vi "Anzahl Span Eingänge Versa Hardware.vi"() -> (3 "Anzahl Span":i32)   [LabVIEW 2020, in "Linearisierung v2.lvlib" / "SpanEinstellungen.lvlib"]
uses:
  SpanEinstellungen.lvlib
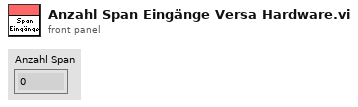
[diagram p1: front panel]
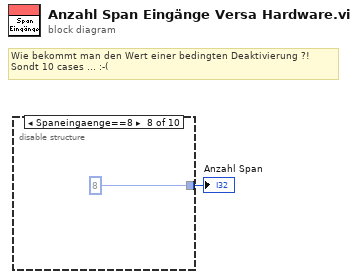
[diagram p0: block diagram]
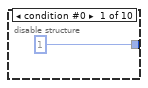
[diagram p2: hidden frame]
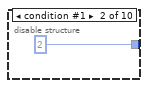
[diagram p3: hidden frame]
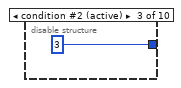
[diagram p4: hidden frame]
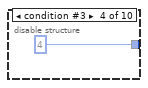
[diagram p5: hidden frame]
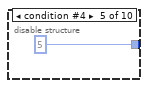
[diagram p6: hidden frame]
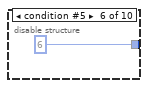
[diagram p7: hidden frame]
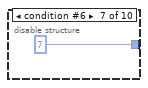
[diagram p8: hidden frame]
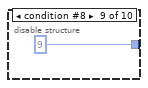
[diagram p9: hidden frame]
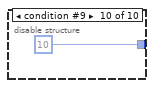
[diagram p10: hidden frame]
diagram:
  # "Wie bekommt man den Wert einer bedingten Deaktivierung ?!\nSondt 10 cases ... :-("
  n1 = disable-structure shown="Spaneingaenge==8" {
    disable-tunnel: [1 ("y") 2 ("y") 3 ("y") 4 ("y") 5 ("y") 6 ("y") 7 ("y") 8 ("y") 9 ("y") 10 ("y")] -> w1
    frame condition #0 {
    }
    frame condition #1 {
    }
    frame condition #2 (active) {
    }
    frame condition #3 {
    }
    frame condition #4 {
    }
    frame condition #5 {
    }
    frame condition #6 {
    }
    frame condition #7 {
    }
    frame condition #8 {
    }
    frame condition #9 {
    }
  }
  "Anzahl Span" <- w1
